vi "Intersperse Data with Invalid Data (multiple channel) complex data.vi"(1 "Intersperse Ratio":dbl=0.1, 5 "Channel0 Input":cdb[](array[numeric]) format="%.16g", 7 "Channel1 Input":cdb[](array[numeric]) format="%.16g") -> (6 "Channel0 Output":cdb[](array[numeric]), 8 "Channel1 Output":cdb[](array[numeric]), 10 "Data Valid":bool[](array[boolean]))   [LabVIEW 2011]
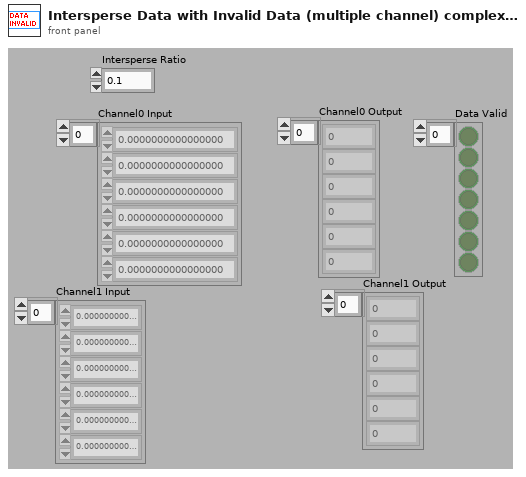
[diagram p1: front panel]
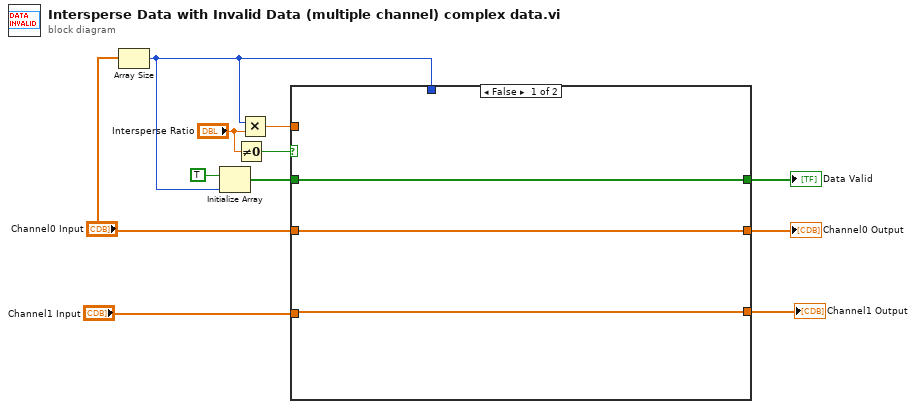
[diagram p0: block diagram]
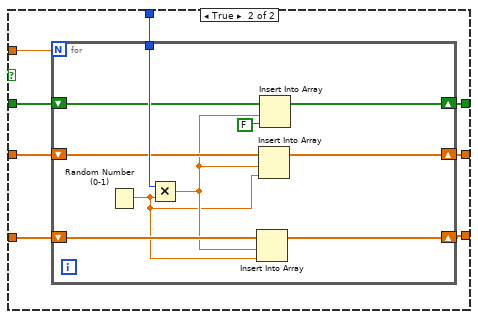
[diagram p2: hidden frame]
diagram:
  n1 = Array Size(array="Channel0 Input") -> (size(s)=w10:i32)
  n2 = Initialize Array(TRUE, w10) -> (w8:bool[])
  n3 = Not Equal To 0?(x="Intersperse Ratio") -> (x != 0?=w1:bool)
  n4 = Multiply(x=w10, y="Intersperse Ratio") -> (x*y=w3:dbl)
  n5 = case shown="False" w1 {
    tunnel: "Channel0 Input" -> [w14 w22]
    tunnel: w10 -> [_ w21]
    tunnel: w8 -> [w13 w20]
    tunnel: [w13 w19] -> w7
    tunnel: [w14 w18] -> w6
    tunnel: "Channel1 Input" -> [w12 w17]
    tunnel: [w12 w16] -> w4
    tunnel: w3 -> [_ w15]
    frame False {
    }
    frame True {
      n6 = for {
        N: w15 -> [_]
        tunnel: w21 -> [w32]
        shift-right: [w30] -> w18
        shift-left: w22 -> [w31]
        shift-right: [w28] -> w19
        shift-left: w20 -> [w29]
        shift-right: [w23] -> w16
        shift-left: w17 -> [w26]
        n7 = Random Number (0-1)() -> (number: 0 to 1=w24:dbl)
        n8 = Multiply(x=w32, y=w24) -> (x*y=w25:dbl)
        n9 = Insert Into Array(array=w26, index=w25, new element=w24) -> (w23:cdb[])
        n10 = Insert Into Array(array=w31, index=w25, new element=w24) -> (w30:cdb[])
        n11 = Insert Into Array(array=w29, index=w25, new element=FALSE) -> (w28:bool[])
      }
    }
  }
  "Data Valid" <- w7
  "Channel0 Output" <- w6
  "Channel1 Output" <- w4
